vi "Add IO Control.vi"(8 "error in (no error)":errorcluster, 11 "Node Ptr":u64 format="%.0x") -> (0 "error out":errorcluster)   [LabVIEW 2015, in "Diagnostics Addon System Explorer.lvlib"]
uses:
  Diagnostics Addon System Explorer.lvlib
  Shared/Types/IO Control Parameters.ctl
  Shared/Types/Input and Output Signal Parameters.ctl
  Shared/Types/Signal Parameters.ctl
  <vilib>/NI Veristand/Custom Device API/Custom Device API.lvlib
  <vilib>/NI Veristand/Custom Device Tools/Custom Device Utility Library/Custom Device Utility Library.lvlib
  Shared/Diagnostics Addon Shared.lvlib
panel:
  in  "Tag":string
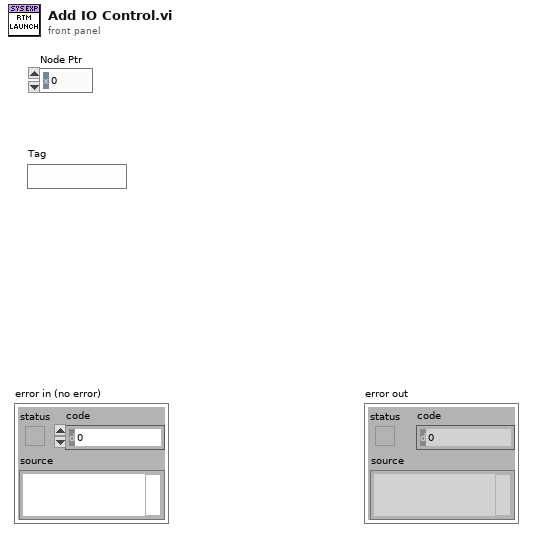
[diagram p1: front panel]
types:
  T1 = typedef "Custom Device API.lvlib/Custom Device Item Ref.ctl" = u64
  T2 = typedef "Custom Device API.lvlib/Custom Device Item Info.ctl" = cluster{"Name":string, "Is Channel":bool, "GUID":string, "Is Waveform":bool}
  T3 = typedef "Diagnostics Addon Shared.lvlib/IO Control Parameters.ctl" = cluster{"Name":string, "Description":string, "ID":u16, "Mode":u8, "Signals":T4}
  T4 = typedef "Diagnostics Addon Shared.lvlib/Input and Output Signal Parameters.ctl" = cluster{"Cmd":T5[], "Response":T5[]}
  T5 = typedef "Diagnostics Addon Shared.lvlib/Signal Parameters.ctl" = cluster{"Start Bit":u8, "Length":u8, "Scaling Factor":dbl, "Scaling Offset":dbl, "Minimum":dbl, "Maximum":dbl, "Data Type":u32, "Byte Order":u32, "Default Value":dbl, "Name":string, "Units":string, "Description":string}
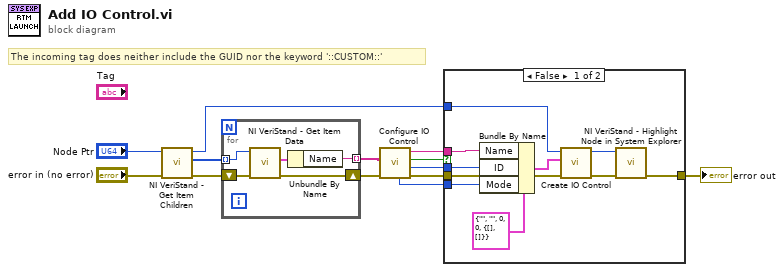
[diagram p0: block diagram]
diagram:
  # "The incoming tag does neither include the GUID nor the keyword '::CUSTOM::'"
  n1 = call <vilib>:"NI VeriStand - Get Item Children.vi"("error in (no error)"="error in (no error)", "Item Ref in"="Node Ptr") -> ("error out"=w11:errorcluster, "Child Refs"=w9:T1[], "Item Ref out"=w8:T1)  [unwired: 6 in, 1 out]
  n2 = for {
    tunnel: [w16] -> w7 mode=indexing
    shift-right: [w15] -> w6
    shift-left: w11 -> [w17]
    tunnel: w9 -> [w14] mode=indexing
    n3 = call <vilib>:"NI VeriStand - Get Item Data.vi"("error in (no error)"=w17, "Item Ref in"=w14) -> ("error out"=w15:errorcluster, "Item Info"=w18:T2)  [unwired: 8 out]
    n4 = Unbundle By Name(w18) -> ("Name"=w16:string)
  }
  n5 = call "Configure IO Control.vi"("error in (no error)"=w6, "Existing PIDs"=w7) -> ("error out"=w5:errorcluster, "ID out"=w2:u16, "Cancel PID?"=w3:bool, "Name out"=w4:string, "Mode out"=w1:u8)  [unwired: 5 in]
  n6 = case shown="False" w3 {
    tunnel: w5 -> [w27 w29]
    tunnel: w8 -> [w24 _]
    tunnel: w4 -> [w22 _]
    tunnel: [w28 w29] -> w10
    tunnel: w2 -> [w21 _]
    tunnel: w1 -> [w19 _]
    frame False {
      n7 = Bundle By Name(cluster=T3 {"Name"="", "Description"="", "ID"=0, "Mode"=0, "Signals"={"Cmd"=[], "Response"=[]}} ("IO Control"), "Name"=w22, "ID"=w21, "Mode"=w19) -> (w20:T3)
      n8 = call "Create IO Control.vi"("error in (no error)"=w27, "IO Control"=w20, "Section Ptr"=w24) -> ("error out"=w26:errorcluster, "Parent Ref out"=w25:T1)  [unwired: 7 in]
      n9 = call <vilib>:"NI VeriStand - Highlight Node in System Explorer.vi"("error in (no error)"=w26, "Item Ref in"=w25) -> ("error out"=w28:errorcluster)  [unwired: 8 in, 1 out]
    }
    frame True {
    }
  }
  "error out" <- w10
